vi "PC_laser_read_cRIO.vi"() -> ()   [LabVIEW 2020]
panel:
  out "DAQ Error":errorcluster
  out "Daigital Outputs":bool[](array[boolean]) caption="Digital Outputs (DAQ)"
  out "cRIO Error":errorcluster
  out "Readouts (V)":T1
  out "Laser Displacement Readings (cRIO)":cluster{dbl, dbl, dbl, dbl}(graph)
  in  "stop":bool
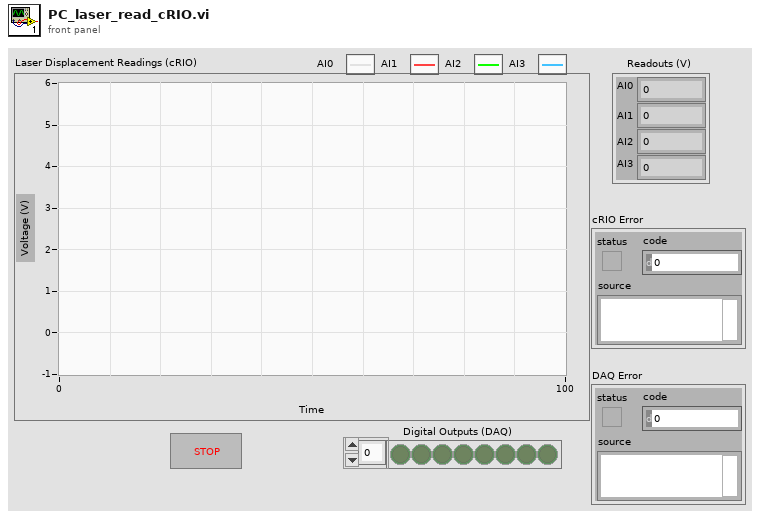
[diagram p1: front panel]
types:
  T1 = cluster{"AI0":dbl, "AI1":dbl, "AI2":dbl, "AI3":dbl}
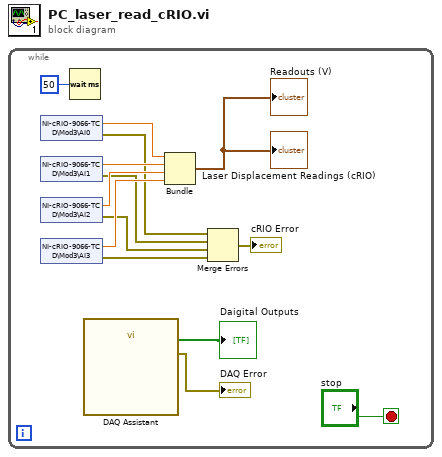
[diagram p0: block diagram]
diagram:
  n1 = while {
    stop <- "stop" stop-if-true
    n2 = shared-variable "NI-cRIO-9066-TCD\\Mod3\\AI0"() -> (w12:dbl, error out=w7:errorcluster)  [unwired: 1 in]
    n3 = shared-variable "NI-cRIO-9066-TCD\\Mod3\\AI1"() -> (w11:dbl, error out=w6:errorcluster)  [unwired: 1 in]
    n4 = shared-variable "NI-cRIO-9066-TCD\\Mod3\\AI2"() -> (w10:dbl, error out=w4:errorcluster)  [unwired: 1 in]
    n5 = shared-variable "NI-cRIO-9066-TCD\\Mod3\\AI3"() -> (w9:dbl, error out=w3:errorcluster)  [unwired: 1 in]
    n6 = Wait (ms)(milliseconds to wait=u32 50) -> ()  [unwired: 1 out]
    n7 = call "DAQ Assistant"() -> ("data"=→"Daigital Outputs":bool[], "error out"=→"DAQ Error":errorcluster)  [unwired: 17 in, 1 out]
    n8 = Bundle(w12, w11, w10, w9) -> (→"Laser Displacement Readings (cRIO)" →"Readouts (V)":cluster{dbl, dbl, dbl, dbl})  [unwired: 1 in]
    n9 = Merge Errors(w7, w6, w4, w3) -> (→"cRIO Error":errorcluster)
  }
